vi "Shutdown.vi"(8 "error in (no error)":errorcluster, 11 "DLP2 in":refnum<class "DLP2.lvclass">) -> (0 "error out":errorcluster, 3 "DLP2 out":refnum<class "DLP2.lvclass">)   [LabVIEW 2022 SP3, in "DLP2.lvclass"]
doc: "Developed by Kevin Thompson\nkevin@thompsonengineering.net\n\nCopyright 2018\nThompson Engineering, LLC"
uses:
  DLP2.lvclass
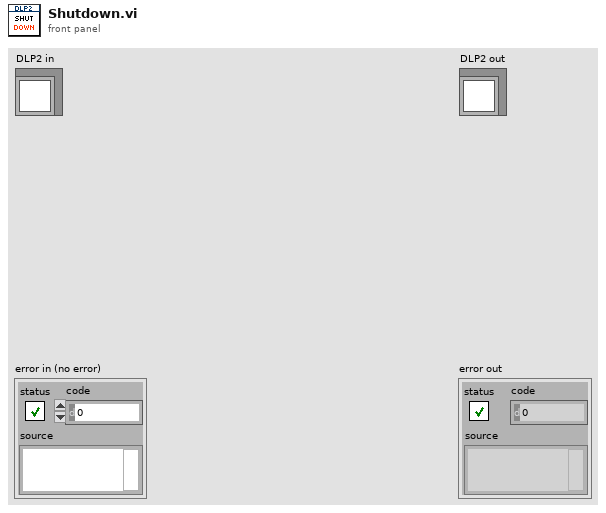
[diagram p1: front panel]
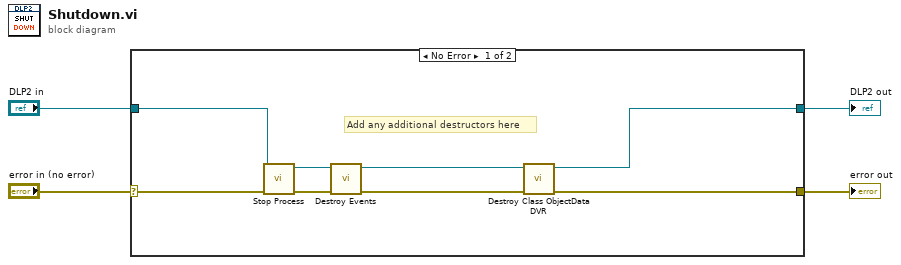
[diagram p0: block diagram]
diagram:
  n1 = case shown="No Error" "error in (no error)" {
    selector: "error in (no error)" -> [w12 w14]
    tunnel: [w7 w14] -> w3
    tunnel: [w5 w13] -> w1
    tunnel: "DLP2 in" -> [w10 w13]
    frame No Error {
      # "Add any additional destructors here"
      n2 = call "Stop Process.vi"("error in (no error)"=w12, "DLP2 in"=w10) -> ("error out"=w11:errorcluster, "DLP2 out"=w9:refnum<class "DLP2.lvclass">)  [unwired: 8 in]
      n3 = call "Destroy Events.vi"("error in (no error)"=w11, "DLP2 in"=w9) -> ("error out"=w8:errorcluster, "DLP2 out"=w6:refnum<class "DLP2.lvclass">)  [unwired: 8 in]
      n4 = call "Destroy Class ObjectData DVR.vi"("error in (no error)"=w8, "DLP2 in"=w6) -> ("error out"=w7:errorcluster, "DLP2 out"=w5:refnum<class "DLP2.lvclass">)  [unwired: 8 in]
    }
    frame Error {
    }
  }
  "error out" <- w3
  "DLP2 out" <- w1
